vi "RecieveAByte.vi"(11 "Digit Signal":bool) -> (0 "Error?":bool, 3 "Char":u8)   [LabVIEW 2013]
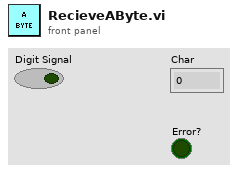
[diagram p1: front panel]
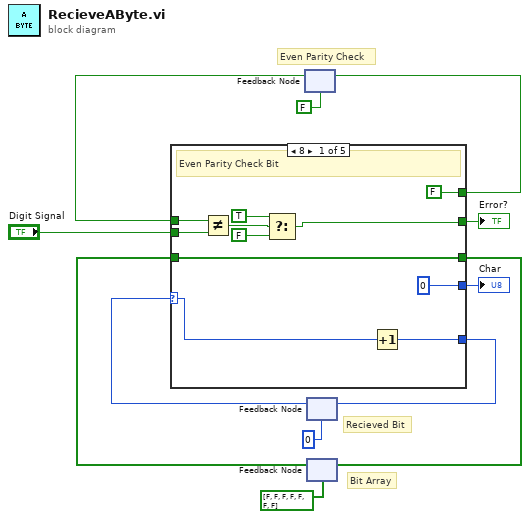
[diagram p0: block diagram]
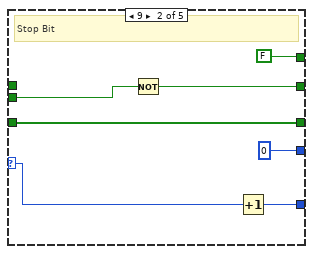
[diagram p2: hidden frame]
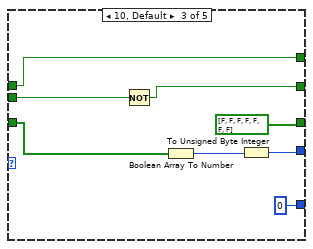
[diagram p3: hidden frame]
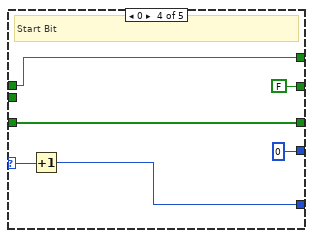
[diagram p4: hidden frame]
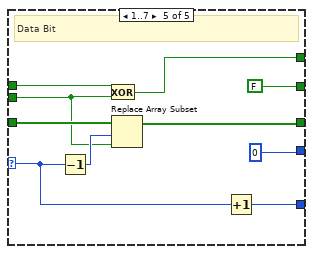
[diagram p5: hidden frame]
diagram:
  # "Recieved Bit"
  # "Bit Array"
  # "Even Parity Check"
  n1 = feedback #1(FALSE) -> (w7:bool)
  n2 = feedback #2(u8 0) -> (w1:i32)
  n3 = feedback #3(bool[] [FALSE, FALSE, FALSE, FALSE, FALSE, FALSE, FALSE]) -> (w6:bool[])
  n4 = case shown="8" w1 {
    selector: w1 -> [w17 w28 _ w40 w46]
    tunnel: "Digit Signal" -> [w20 w24 w32 _ w48]
    tunnel: w6 -> [w15 w27 w34 w42 w50]
    tunnel: [w15 w27 bool[] [FALSE, FALSE, FALSE, FALSE, FALSE, FALSE, FALSE] w42 w51] -> w10
    tunnel: w7 -> [w23 _ w37 w44 w53]
    tunnel: [FALSE FALSE w37 w44 w54] -> w8
    tunnel: [w14 w25 w31 FALSE FALSE] -> w4
    tunnel: [u8 0 u8 0 w35 u8 0 u8 0] -> w5
    tunnel: [w16 w29 u8 0 w39 w45] -> w2
    frame 8 {
      # "Even Parity Check Bit"
      n5 = Not Equal?(x=w23, y=w20) -> (x != y?=w22:bool)
      n6 = Select(t=TRUE, s=w22, f=FALSE) -> (s? t:f=w14:bool)
      n7 = Increment(x=w17) -> (x+1=w16:i32)
    }
    frame 9 {
      # "Stop Bit"
      n8 = Not(x=w24) -> (.not. x?=w25:bool)
      n9 = Increment(x=w28) -> (x+1=w29:i32)
    }
    frame 10, Default {
      n10 = Not(x=w32) -> (.not. x?=w31:bool)
      n11 = Boolean Array To Number(Boolean array=w34) -> (number=w38:u32)
      n12 = To Unsigned Byte Integer(number=w38) -> (unsigned 8bit integer=w35:u8)
    }
    frame 0 {
      # "Start Bit"
      n13 = Increment(x=w40) -> (x+1=w39:i32)
    }
    frame 1..7 {
      # "Data Bit"
      n14 = Decrement(x=w46) -> (x-1=w49:i32)
      n15 = Exclusive Or(1:w48, 2:w53) -> (0:w54:bool)
      n16 = Replace Array Subset(array=w50, new element=w48, index=w49) -> (w51:bool[])
      n17 = Increment(x=w46) -> (x+1=w45:i32)
    }
  }
  "Char" <- w5
  "Error?" <- w4
  n18 = feedback-in #1(w8) -> ()
  n19 = feedback-in #2(w2) -> ()
  n20 = feedback-in #3(w10) -> ()
